vi "Start Measurement.vi"(1 "Acquisition time":i32=1000 min=0 max=3600000 step=1, 2 "DeviceIndex":i32) -> (0 "DataValid":bool)   [LabVIEW 2018]
uses:
  phlib.dll
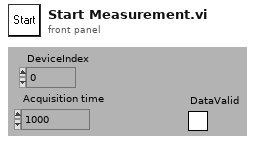
[diagram p1: front panel]
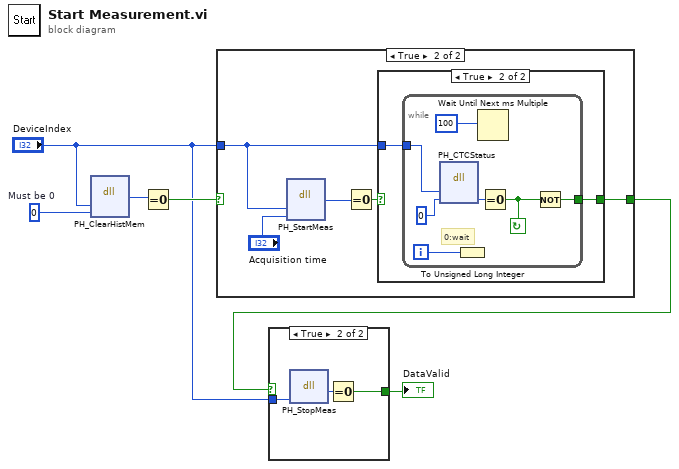
[diagram p0: block diagram]
diagram:
  w2 = u32 0  # Must be 0
  n1 = dll-call lib="phlib.dll" fn="PH_ClearHistMem"("devidx"="DeviceIndex", "block"=w2) -> (w4:i32)  [unwired: 5 in, 2 out]
  n2 = Equal To 0?(x=w4) -> (x = 0?=w3:bool)
  n3 = case shown="True" w3 {
    selector: w3 -> [w7 _]
    tunnel: [w7 w10] -> w6
    tunnel: "DeviceIndex" -> [_ w8]
    frame False {
    }
    frame True {
      n4 = dll-call lib="phlib.dll" fn="PH_StartMeas"("devidx"=w8, "tacq"="Acquisition time") -> (w12:i32)  [unwired: 5 in, 2 out]
      n5 = Equal To 0?(x=w12) -> (x = 0?=w11:bool)
      n6 = case shown="True" w11 {
        selector: w11 -> [w13 _]
        tunnel: [w13 w15] -> w10
        tunnel: w8 -> [_ w14]
        frame False {
        }
        frame True {
          n7 = while {
            tunnel: w14 -> [w18]
            tunnel: [w20] -> w15
            i -> [w19]
            stop <- w21 continue-if-true
            # "0:wait"
            n8 = dll-call lib="phlib.dll" fn="PH_CTCStatus"("devidx"=w18, "ctcstatus"=0) -> ("ctcstatus"=w16:i32)  [unwired: 5 in, 2 out]
            n9 = To Unsigned Long Integer(number=w19) -> ()  [unwired: 1 out]
            n10 = Wait Until Next ms Multiple(millisecond multiple=100) -> ()  [unwired: 1 out]
            n11 = Equal To 0?(x=w16) -> (x = 0?=w21:bool)
            n12 = Not(x=w21) -> (.not. x?=w20:bool)
          }
        }
      }
    }
  }
  n13 = case shown="True" w6 {
    selector: w6 -> [w23 _]
    tunnel: [w23 w25] -> w5
    tunnel: "DeviceIndex" -> [_ w24]
    frame False {
    }
    frame True {
      n14 = dll-call lib="phlib.dll" fn="PH_StopMeas"("devidx"=w24) -> (w26:i32)  [unwired: 4 in, 2 out]
      n15 = Equal To 0?(x=w26) -> (x = 0?=w25:bool)
    }
  }
  "DataValid" <- w5
